vi "NV Global.vi"() -> ()   [LabVIEW 2020]
panel:
  out "new NV":bool
  out "NV Point":dbl[](array[numeric])=[24.65822792285421, -103.77429038112166] format="%.6f"
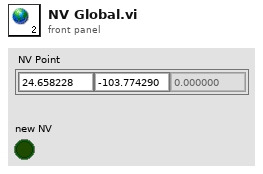
[diagram p1: front panel]
diagram:
